vi "runCopyAll.vi"() -> ()   [LabVIEW 2012]
uses:
  <vilib>/Utility/file.llb/Read From Spreadsheet File (string).vi
panel:
  out "element":string
  out "all rows":string[][](array[string])
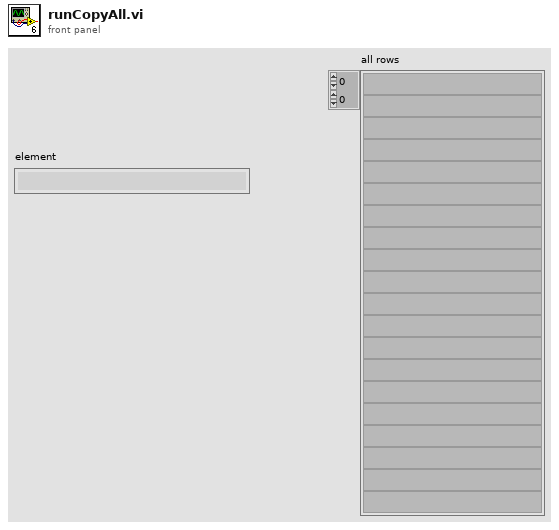
[diagram p1: front panel]
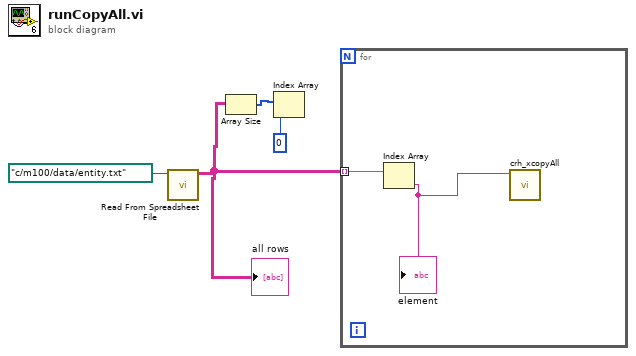
[diagram p0: block diagram]
diagram:
  n1 = call-poly <vilib>:"Read From Spreadsheet File.vi"("file path (dialog if empty)"=path "c:/m100/data/entity.txt") -> ("all rows"=w2:string[][])  [unwired: 6 in, 4 out]
  "all rows" <- w2
  n2 = Array Size(array=w2) -> (size(s)=w4:i32[])
  n3 = Index Array(array=w4, index=0) -> ()  [unwired: 1 out]
  n4 = for {
    tunnel: w2 -> [w6] mode=indexing
    n5 = Index Array(array=w6) -> (element=w5:string)  [unwired: 1 in]
    "element" <- w5
    n6 = call "crh_xcopyAll.vi"("folder"=w5) -> ()  [unwired: 11 in]
  }
